vi "AlliGator Display Current Decay Fit Parameter Map (X,Y, I).vi"(7 "Decay Fit Map Ctrl Refums":T1, 8 "error in (no error)":errorcluster, 11 "AlliGator Internal Variables DVR":refnum<data-value>) -> (0 "error out":errorcluster, 3 "AlliGator Internal Variables DVR":refnum<data-value>)   [LabVIEW 2021, in "AlliGator Action Engine.lvlib"]
doc: "Displays last mouse position and true decay fit parameter map value at that location."
uses:
  Action Engine/AlliGator Action Engine.lvlib
  AlliGator Decay Fit Map Control Refnums.ctl
  Fits/IRF(X)PSED/Decay Fit Parameters & Derived Quantities List v2.ctl
  Internal Variables/AlliGator Internal Variables v2.ctl
  <vilib>/vision/Image Controls.llb/IMAQ Image.ctl
  Internal Variables/AlliGator Gate Image Set.ctl
  Files/AlliGator FLI Dataset Type.ctl
  Files/AlliGator Data Series Type.ctl
  Dual-Channel Datasets/AlliGator Dataset Channel.ctl
  Settings/AlliGator Gate Arithmetic.ctl
  Source Image/AlliGator Displayed Image.ctl
  Image/Named ROI Description.ctl
  Phasor Graph/AlliGator Decay Metadata v3.ctl
  Decay Analysis/Decay Preprocessing/AlliGator Decay Background Subtraction Info.ctl
  Decay Analysis/Decay Preprocessing/AlliGator Baseline Subtraction Method.ctl
  Graphs/XY Graph/XY Graph Plot Shift Parameters.ctl
  Graphs/XY Graph/XY Graph Plot Shift Method.ctl
  Decay Analysis/Decay Preprocessing/AlliGator Decay Extrapolation Parameters.ctl
  Phasor/Calibration Phasor (m, phi).ctl
  Phasor/Phasor Reference Series.ctl
  Phasor/Phasor Calibration Map v2.ctl
  Phasor/Phasor (g, s).ctl
  Phasor Graph/AlliGator Raw Phasor Plot Data v5.ctl
  Phasor/Phasor Standard Deviation Options.ctl
  Phasor Plot/AlliGator Phasor Multi-Harmonic Data.ctl
  Phasor/Phasor Harmonic Data.ctl
  AlliGator Decay Fit Options & Parameters v3.ctl
  Fits/IRF(X)PSED/Decay Fit Options v3.ctl
  Fits/Decay Convolution/Decay Model.ctl
  Fits/Residual Type.ctl
  Fits/IRF(X)PSED/Fit Weights Type.ctl
  Fits/Non-linear Fitting Method v2.ctl
  Fits/Fit Calculation Method.ctl
  Fits/Non-linear Fitting Algorithm.ctl
  Decay Analysis/Decay Fit/AlliGator Decay Fit Parameter Constraints 2.ctl
  Fits/IRF(X)PSED/Decay Fit Parameters In List.ctl
  Fits/IRF(X)PSED/MLE Baseline Offset Type.ctl
  Decay Analysis/Decay Preprocessing/AlliGator Decay Preprocessing Parameters.ctl
  Fits/IRF(X)PSED/Decay Fit Result Constraint.ctl
  AlliGator Parameter Maps Data.ctl
  <vilib>/vision/NI_Vision_Development_Module.lvlib
  AlliGator Decay Fit Parameter Map.lvlib
  Fits/Fits.lvlib
  Phasor/Phasor.lvlib
  Image/Image.lvlib
  Decay Analysis/Decay Preprocessing/AlliGator Decay Preprocessing.lvlib
  Graphs/XY Graph/XY Graph Add-Ons.lvlib
  Phasor Graph/AlliGator Phasor Graph.lvlib
  Files/AlliGator Files.lvlib
  Internal Variables/AlliGator Internal Variables.lvlib
  Phasor Plot/AlliGator Phasor Plot.lvlib
  Source Image/AlliGator Source Image.lvlib
  Decay Analysis/Decay Fit/AlliGator Decay Fit.lvlib
  Settings/AlliGator Settings.lvlib
  Dual-Channel Datasets/AlliGator Dual-Channel Datasets.lvlib
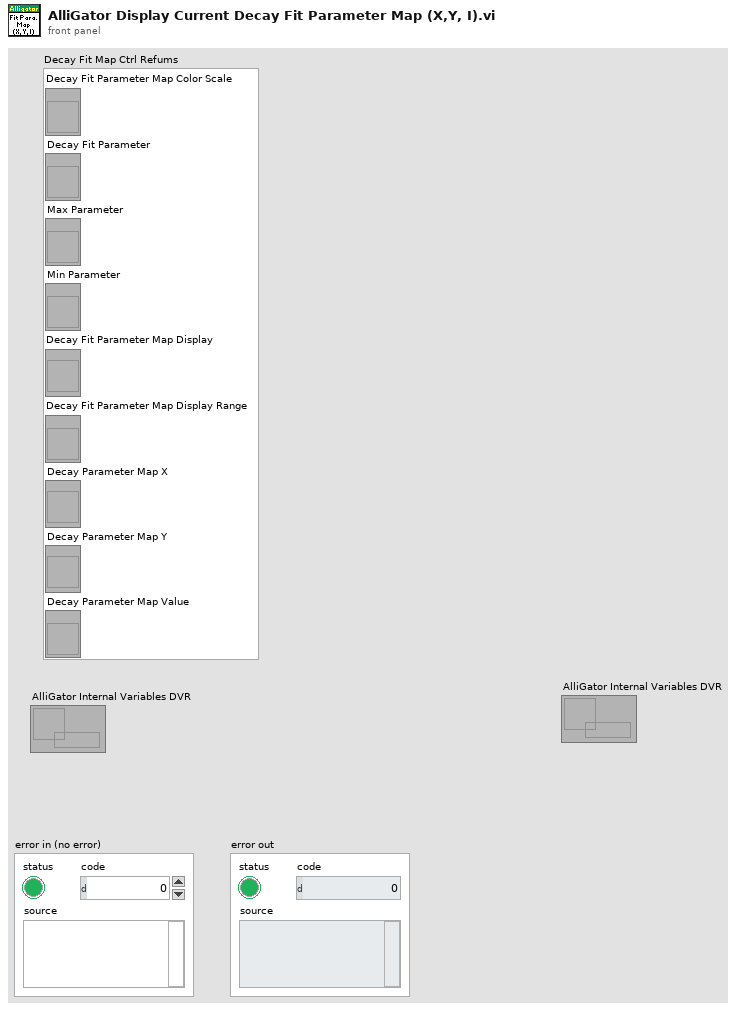
[diagram p1: front panel]
types:
  T1 = typedef "AlliGator Decay Fit Parameter Map.lvlib/AlliGator Decay Fit Map Control Refnums.ctl" = cluster{"Decay Fit Parameter Map Color Scale":refnum<vi>, "Decay Fit Parameter":refnum<vi>, "Max Parameter":refnum<vi>, "Min Parameter":refnum<vi>, "Decay Fit Parameter Map Display":refnum<vi>, "Decay Fit Parameter Map Display Range":refnum<vi>, "Decay Parameter Map X":refnum<vi>, "Decay Parameter Map Y":refnum<vi>, "Decay Parameter Map Value":refnum<vi>}
  T2 = typedef "IMAQ Image.ctl" = refnum<image>
  T3 = typedef "Fits.lvlib/Decay Fit Parameters & Derived Quantities List v2.ctl" = enum16{"Offset", "Baseline", "A_1", "tau_1", "A_2", "tau_2", "<tau>_a", "f1_a", "f2_a", "<tau>_i", "f1_i", "f2_i", "-", "R^2", "Chi^2"}
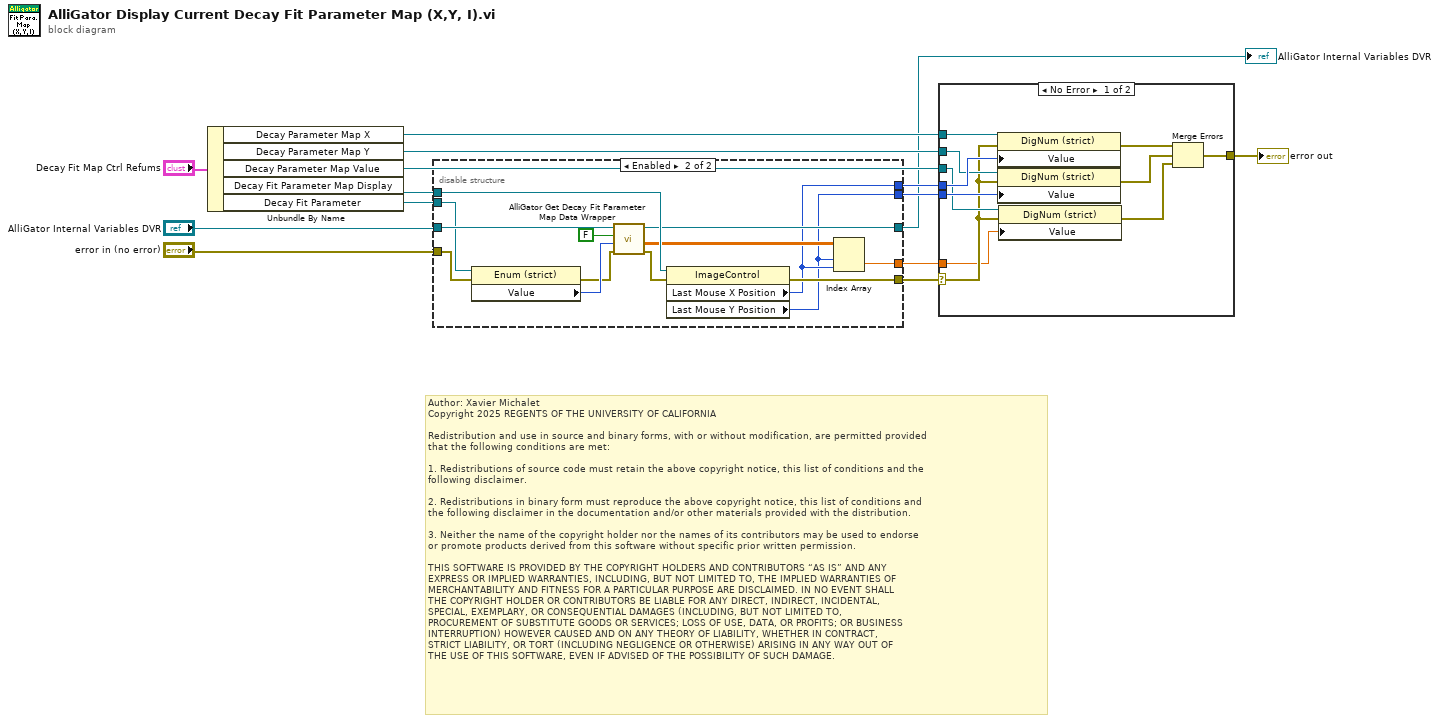
[diagram p0: block diagram]
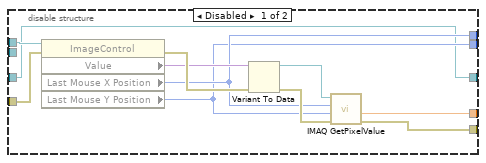
[diagram p2: hidden frame]
diagram:
  # "Author: Xavier Michalet\nCopyright 2025 REGENTS OF THE UNIVERSITY OF CALIFORNIA\n\nRedistribution and use in source and binary forms, with or without modification, are permitted provided\nthat the following conditions are met:\n\n1. Redistributions of source code must retain the above copyright notice, this list of conditions and the\nfollowing disclaimer.\n\n2. Redistributions in binary form must reproduce the above copyright notice, this list of conditions and\nthe following disclaimer in the documentation and/or other materials provided with the distribution.\n\n3. Neither the name of the copyright holder nor the names of its contributors may be used to endorse \nor promote products derived from this software without specific prior written permission.\n\nTHIS SOFTWARE IS PROVIDED BY THE COPYRIGHT HOLDERS AND CONTRIBUTORS “AS IS” AND ANY \nEXPRESS OR IMPLIED WARRANTIES, INCLUDING, BUT NOT LIMITED TO, THE IMPLIED WARRANTIES OF\nMERCHANTABILITY AND FITNESS FOR A PARTICULAR PURPOSE ARE DISCLAIMED. IN NO EVENT SHALL\nTHE COPYRIGHT HOLDER OR CONTRIBUTORS BE LIABLE FOR ANY DIRECT, INDIRECT, INCIDENTAL, \nSPECIAL, EXEMPLARY, OR CONSEQUENTIAL DAMAGES (INCLUDING, BUT NOT LIMITED TO, \nPROCUREMENT OF SUBSTITUTE GOODS OR SERVICES; LOSS OF USE, DATA, OR PROFITS; OR BUSINESS\nINTERRUPTION) HOWEVER CAUSED AND ON ANY THEORY OF LIABILITY, WHETHER IN CONTRACT, \nSTRICT LIABILITY, OR TORT (INCLUDING NEGLIGENCE OR OTHERWISE) ARISING IN ANY WAY OUT OF\nTHE USE OF THIS SOFTWARE, EVEN IF ADVISED OF THE POSSIBILITY OF SUCH DAMAGE."
  n1 = Unbundle By Name("Decay Fit Map Ctrl Refums") -> ("Decay Parameter Map X"=w11:refnum<vi>, "Decay Parameter Map Y"=w9:refnum<vi>, "Decay Parameter Map Value"=w7:refnum<vi>, "Decay Fit Parameter Map Display"=w12:refnum<vi>, "Decay Fit Parameter"=w3:refnum<vi>)
  n2 = disable-structure shown="Enabled" {
    disable-tunnel: "error in (no error)" -> [w21 w36]
    disable-tunnel: w12 -> [w20 w38]
    disable-tunnel: [w19 w30] -> w10
    disable-tunnel: [w18 w29] -> w8
    disable-tunnel: [w17 w31] -> w6
    disable-tunnel: "AlliGator Internal Variables DVR" -> [w15 w39]
    disable-tunnel: w3 -> [_ w37]
    disable-tunnel: [w15 w34] -> w2
    disable-tunnel: [w16 w32] -> w1
    frame Disabled {
      n3 = property class="ImageControl"(reference=w20, error in=w21) -> (error out=w24:errorcluster, "Value"=w22:variant, "Last Mouse X Position"=w19:i32, "Last Mouse Y Position"=w18:i32)  [unwired: 1 out]
      n4 = Variant To Data(error in=w24, Variant=w22) -> (data=w23:T2, error out=w25:errorcluster)  [unwired: 1 in]
      n5 = call "IMAQ GetPixelValue"("Image"=w23, "X Coordinate"=w19, "Y Coordinate"=w18, "error in (no error)"=w25) -> ("Pixel Value (Float)"=w16:sgl, "error out"=w17:errorcluster)  [unwired: 2 in, 3 out]
    }
    frame Enabled {
      n6 = property class="Enum (strict)"(reference=w37, error in=w36) -> (error out=w27:errorcluster, "Value"=w35:T3)  [unwired: 1 out]
      n7 = call "AlliGator Get Decay Fit Parameter Map Data Wrapper.vi"("error in (no error)"=w27, "Fit Parameter"=w35, "Compute Decay Fit Parameter Map"=FALSE, "Data Value Reference in"=w39) -> ("error out"=w26:errorcluster, "Map Data"=w33:dbl[][], "Data Value Reference out"=w34:refnum<data-value>)  [unwired: 2 in, 3 out]
      n8 = property class="ImageControl"(reference=w38, error in=w26) -> (error out=w31:errorcluster, "Last Mouse X Position"=w30:i32, "Last Mouse Y Position"=w29:i32)  [unwired: 1 out]
      n9 = Index Array(array=w33, index (row)=w29, index (col)=w30) -> (element=w32:dbl)
    }
  }
  "AlliGator Internal Variables DVR" <- w2
  n10 = case shown="No Error" w6 {
    selector: w6 -> [w45 _]
    tunnel: w11 -> [w50 _]
    tunnel: w10 -> [w49 _]
    tunnel: w9 -> [w48 _]
    tunnel: w8 -> [w47 _]
    tunnel: w7 -> [w46 _]
    tunnel: [w41 _] -> w5
    tunnel: w1 -> [w40 _]
    frame No Error {
      n11 = property class="DigNum (strict)"(reference=w50, error in=w45, "Value"=w49) -> (error out=w44:errorcluster)  [unwired: 1 out]
      n12 = property class="DigNum (strict)"(reference=w48, error in=w45, "Value"=w47) -> (error out=w43:errorcluster)  [unwired: 1 out]
      n13 = property class="DigNum (strict)"(reference=w46, error in=w45, "Value"=w40) -> (error out=w42:errorcluster)  [unwired: 1 out]
      n14 = Merge Errors(w44, w43, w42) -> (w41:errorcluster)
    }
    frame Error {
      # "Not an image: map is not available"
    }
  }
  "error out" <- w5
